vi "Write  Delay (µs).vi"(8 "error in (no error)":errorcluster, 10 "Delay (µs)":dbl min=0.0 max=100000000.0 format="%.4f", 11 "BME_DG_Chnl in":refnum<class "BME_DG_Chnl.lvclass">) -> (0 "error out":errorcluster, 3 "BME_DG_Chnl out":refnum<class "BME_DG_Chnl.lvclass">)   [LabVIEW 2009, in "POLARIS BME DG.lvlib" / "BME_DG_Chnl.lvclass"]
uses:
  BME_DG_Chnl.lvclass
  BME_DG_Chnl.lvclass/BME_DG_Chnl.ctl
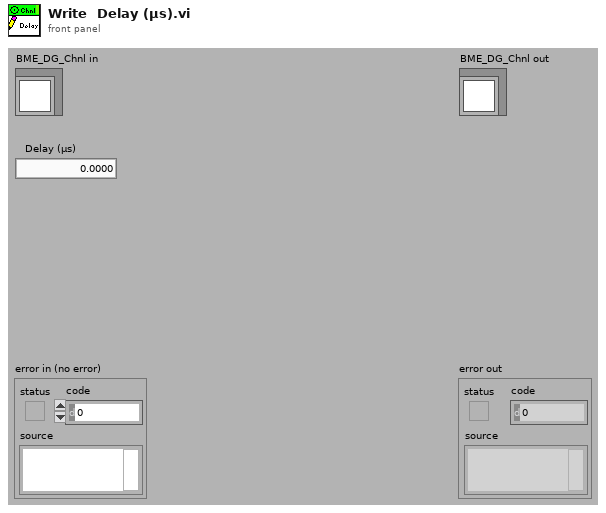
[diagram p1: front panel]
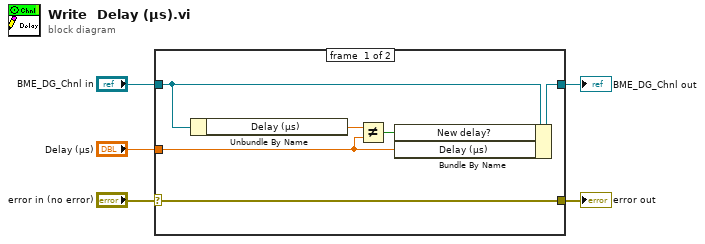
[diagram p0: block diagram]
diagram:
  n1 = case shown="No Error" "error in (no error)" {
    selector: "error in (no error)" -> [w11 w12]
    tunnel: [w11 w12] -> w4
    tunnel: [w10 w13] -> w2
    tunnel: "BME_DG_Chnl in" -> [w9 w13]
    tunnel: "Delay (µs)" -> [w7 _]
    frame #0 {
      n2 = Unbundle By Name(w9) -> ("Delay (µs)"=w8:dbl)
      n3 = Not Equal?(x=w8, y=w7) -> (x != y?=w6:bool)
      n4 = Bundle By Name(cluster=w9, "New delay?"=w6, "Delay (µs)"=w7) -> (w10:refnum<class "BME_DG_Chnl.lvclass">)
    }
    frame #1 {
    }
  }
  "error out" <- w4
  "BME_DG_Chnl out" <- w2
